vi "Init LaunchPad.vi"(8 "error in":errorcluster, 10 "Baud Rate (9600)":u32=9600, 11 "VISA resource":refnum<visa-resource-name>) -> (0 "error out":errorcluster, 3 "VISA resource name out":refnum<visa-resource-name>)   [LabVIEW 2011]
doc: "Initializes a connection to an Arduino running the LabVIEW Interface for Arduino sketch.\n\nNote: The baud rate specified must match the baud rate defined by DEFAULTBAUDRATE in the Arduino firmware.\n\nNote: The Bytes Per Packet input must match the COMMANDLENGTH specified in the Arduino firmware."
uses:
  <vilib>/Instr/_visa.llb/VISA Configure Serial Port (Instr).vi
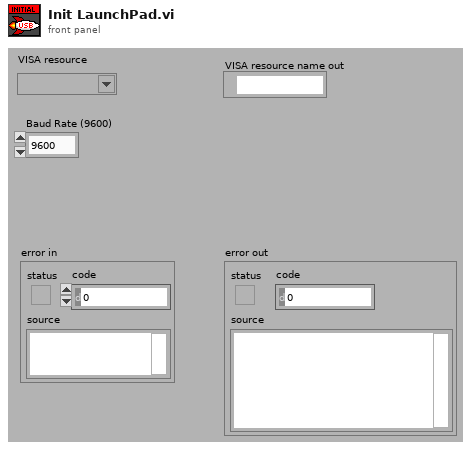
[diagram p1: front panel]
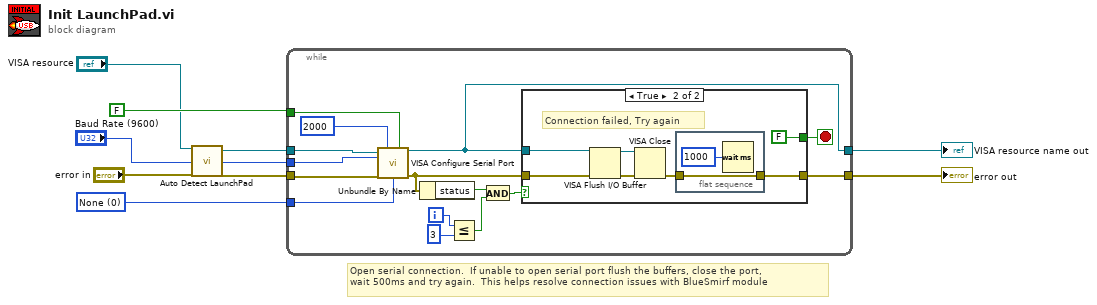
[diagram p0: block diagram]
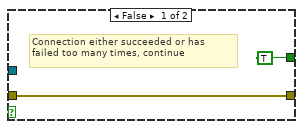
[diagram p2: hidden frame]
diagram:
  w9 = u16 0 items=["None", "XON/XOFF", "RTS/CTS", "XON/XOFF & RTS/CTS", "DTR/DSR", "XON/XOFF & DTR/DSR"] ("flow control (0:none)")
  # "Open serial connection.  If unable to open serial port flush the buffers, close the port,\nwait 500ms and try again.  This helps resolve connection issues with BlueSmirf module"
  n1 = call "Auto Detect LaunchPad.vi"("Visa Resource"="VISA resource", "error in (no error)"="error in") -> ("VISA resource"=w4:refnum<visa-resource-name>, "error out"=w1:errorcluster)  [unwired: 12 in]
  n2 = while {
    tunnel: w9 -> [w24]
    tunnel: FALSE ("Enable Termination\nChar (T)") -> [w23]
    tunnel: "Baud Rate (9600)" -> [w22]
    tunnel: w4 -> [w11]
    tunnel: [w15] -> w5
    tunnel: [w13] -> w6
    tunnel: w1 -> [w10]
    i -> [w20]
    stop <- w14 stop-if-true
    n3 = call-poly "VISA Configure Serial Port"("VISA resource name"=w11, "timeout (10sec)"=u32 2000, "Enable Termination\nChar (T)"=w23, "baud rate (9600)"=w22, "error in (no error)"=w10, "flow control (0:none)"=w24) -> ("VISA resource name out"=w13:refnum<visa-resource-name>, "error out"=w16:errorcluster)  [unwired: 8 in]
    n4 = Unbundle By Name(w16) -> ("status"=w18:bool)
    n5 = Less Or Equal?(x=w20, y=3) -> (x <= y?=w19:bool)
    n6 = And(x=w18, y=w19) -> (x .and. y?=w17:bool)
    n7 = case shown="True" w17 {
      tunnel: w16 -> [w26 w29]
      tunnel: [w26 w28] -> w15
      tunnel: [TRUE FALSE] -> w14
      tunnel: w13 -> [_ w32]
      frame False {
        # "Connection either succeeded or has \nfailed too many times, continue"
      }
      frame True {
        # "Connection failed, Try again"
        n8 = VISA Flush I/O Buffer(VISA resource name=w32, error in (no error)=w29) -> (VISA resource name out=w31:refnum<visa-resource-name>, error out=w30:errorcluster)  [unwired: 1 in]
        n9 = VISA Close(VISA resource name=w31, error in (no error)=w30) -> (error out=w27:errorcluster)
        n10 = flat-sequence {
          tunnel: [w34] -> w28
          tunnel: w27 -> [w34]
          frame #0 {
            n11 = Wait (ms)(milliseconds to wait=u32 1000) -> ()  [unwired: 1 out]
          }
        }
      }
    }
  }
  "VISA resource name out" <- w6
  "error out" <- w5
